vi "Initialize VIs Communication.vi"(8 "error in (no error)":errorcluster, 11 "Channel in":refnum<class "Channel.lvclass">) -> (0 "error out":errorcluster, 3 "Channel out":refnum<class "Channel.lvclass">)   [LabVIEW 2018, in "Channel.lvclass"]
doc: "Initialze the communcation with S4GUI"
uses:
  Channel.lvclass
  Channel.lvclass/Channel.ctl
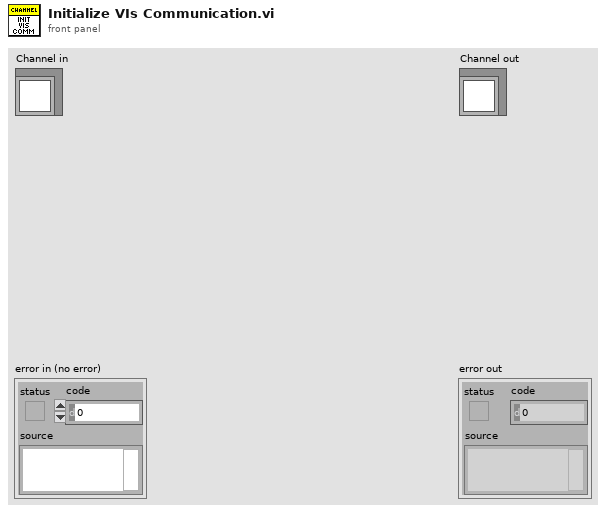
[diagram p1: front panel]
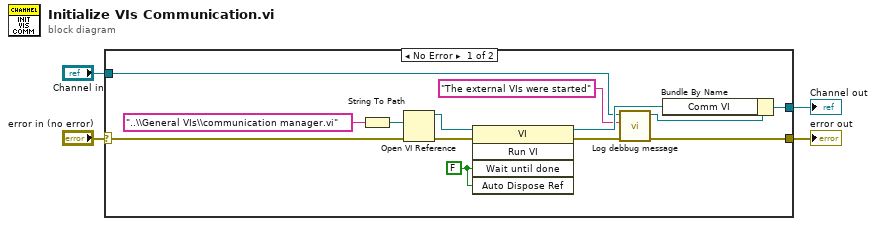
[diagram p0: block diagram]
diagram:
  n1 = case shown="No Error" "error in (no error)" {
    selector: "error in (no error)" -> [w17 w19]
    tunnel: [w8 w19] -> w3
    tunnel: [w16 w18] -> w1
    tunnel: "Channel in" -> [w7 w18]
    frame No Error {
      w13 = FALSE ("Wait Until Done")
      n2 = String To Path(string="..\\General VIs\\communication manager.vi" ("name or relative path")) -> (path=w14:path)
      n3 = Open VI Reference(vi path=w14, error in (no error)=w17) -> (vi reference=w12:refnum<vi>, error out=w15:errorcluster)  [unwired: 4 in]
      n4 = invoke class="VI" method="Run VI"(reference=w12, error in=w15, "Wait until done"=w13, "Auto Dispose Ref"=w13) -> (reference out=w10:refnum<vi>, error out=w9:errorcluster)  [unwired: 1 in, 3 out]
      n5 = call "Log debbug message.vi"("error in (no error)"=w9, "String"="The external VIs were started", "Channel in"=w7) -> ("error out"=w8:errorcluster, "Channel out"=w6:refnum<class "Channel.lvclass">)  [unwired: 7 in]
      n6 = Bundle By Name(cluster=w6, "Comm VI"=w10) -> (w16:refnum<class "Channel.lvclass">)
    }
    frame Error {
    }
  }
  "error out" <- w3
  "Channel out" <- w1
